vi "Example.vi"() -> ()   [LabVIEW 2019]
uses:
  SubModules/FPGA Addon Speciality IO/Source/Types/PWM.Measure.Digital.Measurement.ctl
  SubModules/FPGA Addon Speciality IO/Source/Types/PWM.Measure.Digital.Result.ctl
  SubModules/FPGA Addon Speciality IO/Source/Types/PWM.Generate.Digital.Convert.Settings.ctl
  SubModules/FPGA Addon Speciality IO/Source/Types/PWM.Generate.Digital.Settings.ctl
  SubModules/FPGA Addon Speciality IO/Source/Types/PWM.Measure.Analog.Measurement.ctl
  SubModules/FPGA Addon Speciality IO/Source/Types/PWM.Measure.Analog.Result.ctl
  SubModules/FPGA Addon Speciality IO/Source/Types/PWM.Measure.Digital.Settings.ctl
  SubModules/FPGA Addon Speciality IO/Source/Types/PWM.Measure.Analog.Settings.ctl
  SubModules/FPGA Addon Speciality IO/Source/Types/Sine.Generate.Settings.ctl
  SubModules/FPGA Addon Speciality IO/Source/Types/Sine.Generate.Convert.Settings.ctl
  <vilib>/Platform/TimedLoop/XDataNode/timing_clust.ctl
  <vilib>/Platform/TimedLoop/XDataNode/nitl_modes.ctl
  <vilib>/Platform/TimedLoop/XDataNode/wakeup.ctl
  <vilib>/Platform/TimedLoop/XDataNode/XDataNode.xnode
  SubModules/FPGA Addon Speciality IO/Source/Speciality FPGA IO.lvlib
  <vilib>/Platform/TimedLoop/XDataNode/XDNodeRunTimeDep.lvlib
panel:
  out "Generation.Sine.Ticks":u32
  in  "Generatie.Sine.Ch1.Settings":T1={"AMP"=10.0, "OFFSET"=0.0, "FREQ"=2000.0}
  in  "Generatie.Sine.Ch0.Settings":T1={"AMP"=1.0, "OFFSET"=0.0, "FREQ"=1000.0}
  out "Generate.Sine.Ch1.Internal.Settings":T2={"AMP"=0.0, "OFFSET"=0.0, "PERIODS/TICKS"=0.0002500000409781933}
  out "Generate.Sine.Chl0.Internal.Settings":T2={"AMP"=0.0, "OFFSET"=0.0, "PERIODS/TICKS"=0.0002500000409781933}
  out "Generate.Sine.Convert.Ticks":u32=84
  in  "Sine":bool=TRUE
  out "PWM1":fxp<+/-,32,8>=11.7987060546875
  out "PWM0":fxp<+/-,32,8>=-12.2012939453125
  out "Generate.Digital.Ticks":u32=114
  out "Measure.Digital.Ticks":u32=84
  out "Measure.Analog.Ticks":u32=84
  in  "Measure.Analog.Ch1.Settings":T3={"ACTIVE EDGE"=FALSE, "TIMEOUT"=40000000, "THRESHOLD"=95.0}
  in  "Measure.Analog.Ch0.Settings":T3={"ACTIVE EDGE"=TRUE, "TIMEOUT"=40000000, "THRESHOLD"=0.0}
  in  "Measure.Digital.Ch1.Settings":T4={"ACTIVE EDGE"=FALSE, "TIMEOUT"=40000000}
  in  "Measure.Digital.Ch0.Settings":T4={"ACTIVE EDGE"=TRUE, "TIMEOUT"=40000000}
  out "Measure.Analog.Analyzed":T5[](array[typedef])=[{"FREQ"=5000.0, "PERIOD"=0.00020000001, "DC"=50.0, "ACTIVE TIME"=0.000100000005, "ACTIVE VOLTAGE"=4.979252, "INACTIVE VOLTAGE"=-4.9794044}, {"FREQ"=999.99994, "PERIOD"=0.001, "DC"=90.0, "ACTIVE TIME"=0.0009, "ACTIVE VOLTAGE"=-6.998723, "INACTIVE VOLTAGE"=6.9985094}]
  out "Measure.Analog.Ch1.Results":T6={"ACTIVE TICKS"=90, "INACTIVE TICKS"=10, "ACQ TICKS"=400, "ACTIVE VOLTAGE"=-6.998723030090332, "INACTIVE VOLTAGE"=6.998509407043457}
  out "Measure.Analog.Ch0.Results":T6={"ACTIVE TICKS"=10, "INACTIVE TICKS"=10, "ACQ TICKS"=400, "ACTIVE VOLTAGE"=4.979251861572266, "INACTIVE VOLTAGE"=-4.979404449462891}
  out "Generate.Digital.Ch1.Internal.Settings":T7={"ACTIVE EDGE"=FALSE, "ACTIVE TICKS"=60000000, "INACTIVE TICKS"=20000000}
  out "Generate.Digital.Ch0.Internal.Settings":T7={"ACTIVE EDGE"=TRUE, "ACTIVE TICKS"=4000, "INACTIVE TICKS"=12000}
  in  "Generate.Digital.Channel0.Settings":T8={"ACTIVE EDGE"=FALSE, "FREQ"=0.5, "DC"=50.0}
  in  "Generate.Digital.Channel0.Settings":T8={"ACTIVE EDGE"=TRUE, "FREQ"=2500.0, "DC"=25.0}
  out "Measure.Digital.Analyzed":T9[](array[typedef])=[{"FREQ"=2500.0, "PERIOD"=0.00040000002, "DC"=25.0, "ACTIVE TIME"=0.000100000005}, {"FREQ"=0.0, "PERIOD"=0.0, "DC"=0.0, "ACTIVE TIME"=0.0}]
  out "Measure.Digital.Ch1.Results":T10
  out "Measure.Digital.Ch0.Results":T10={"ACTIVE TICKS"=4000, "INACTIVE TICKS"=12000, "ACQ TICKS"=1}
  in  "Generation.Sine.Ticks":u32=10 caption="Loop Rate"
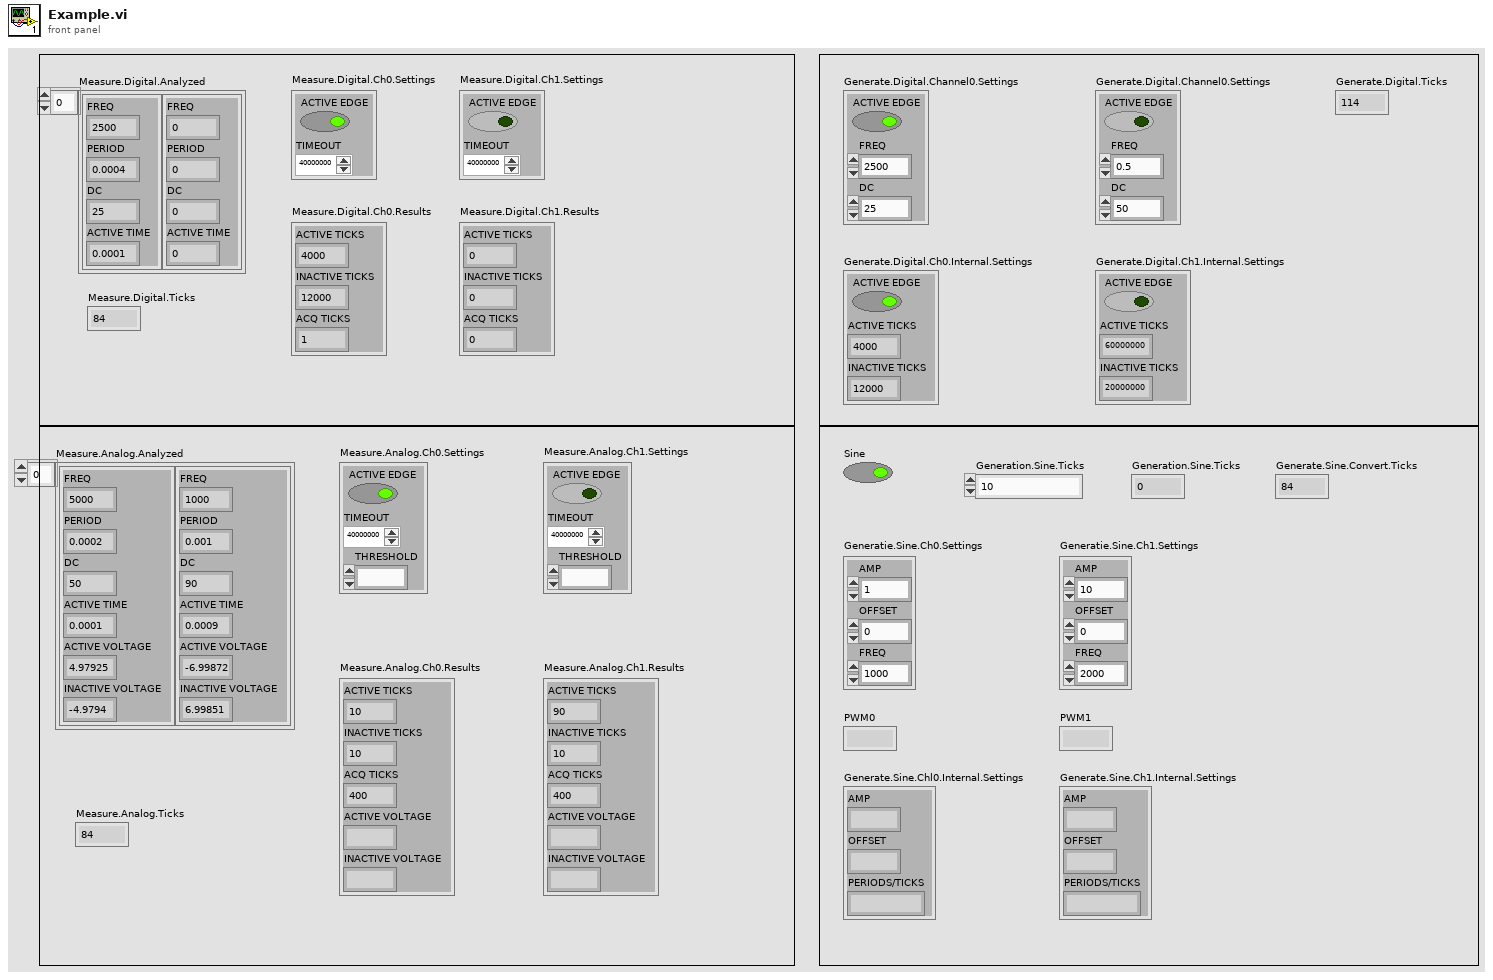
[diagram p1: front panel]
types:
  T1 = typedef "Speciality FPGA IO.lvlib/Sine.Generate.Convert.Settings.ctl" = cluster{"AMP":sgl, "OFFSET":sgl, "FREQ":sgl}
  T2 = typedef "Speciality FPGA IO.lvlib/Sine.Generate.Settings.ctl" = cluster{"AMP":fxp<+/-,32,8>, "OFFSET":fxp<+/-,32,8>, "PERIODS/TICKS":fxp<+,32,0>}
  T3 = typedef "Speciality FPGA IO.lvlib/PWM.Measure.Analog.Settings.ctl" = cluster{"ACTIVE EDGE":bool, "TIMEOUT":u32, "THRESHOLD":fxp<+/-,32,8>}
  T4 = typedef "Speciality FPGA IO.lvlib/PWM.Measure.Digital.Settings.ctl" = cluster{"ACTIVE EDGE":bool, "TIMEOUT":u32}
  T5 = typedef "Speciality FPGA IO.lvlib/PWM.Measure.Analog.Result.ctl" = cluster{"FREQ":sgl, "PERIOD":sgl, "DC":sgl, "ACTIVE TIME":sgl, "ACTIVE VOLTAGE":sgl, "INACTIVE VOLTAGE":sgl}
  T6 = typedef "Speciality FPGA IO.lvlib/PWM.Measure.Analog.Measurement.ctl" = cluster{"ACTIVE TICKS":u32, "INACTIVE TICKS":u32, "ACQ TICKS":u32, "ACTIVE VOLTAGE":fxp<+/-,32,8>, "INACTIVE VOLTAGE":fxp<+/-,32,8>}
  T7 = typedef "Speciality FPGA IO.lvlib/PWM.Generate.Digital.Settings.ctl" = cluster{"ACTIVE EDGE":bool, "ACTIVE TICKS":u32, "INACTIVE TICKS":u32}
  T8 = typedef "Speciality FPGA IO.lvlib/PWM.Generate.Digital.Convert.Settings.ctl" = cluster{"ACTIVE EDGE":bool, "FREQ":sgl, "DC":sgl}
  T9 = typedef "Speciality FPGA IO.lvlib/PWM.Measure.Digital.Result.ctl" = cluster{"FREQ":sgl, "PERIOD":sgl, "DC":sgl, "ACTIVE TIME":sgl}
  T10 = typedef "Speciality FPGA IO.lvlib/PWM.Measure.Digital.Measurement.ctl" = cluster{"ACTIVE TICKS":u32, "INACTIVE TICKS":u32, "ACQ TICKS":u32}
  T11 = typedef "XDNodeRunTimeDep.lvlib/timing_clust.ctl" = cluster{"Expected End [f-1]":u64, "Actual End [f-1]":u64, "Finished Late? [f-1]":bool, "Expected End [i-1]":u64, "Actual End [i-1]":u64, "Finished Late? [i-1]":bool, "Expected Start [i]":u64, "Actual Start [i]":u64, "Expected Start [f]":u64, "Actual Start [f]":u64, "Source Name":string, "Structure Name":string, "Period":i64, "Deadline":i64, "Offset":i64, "Start":i64, "Priority":i32, "Timeout":i32, "Mode":T12, "Wakeup Reason":T13, "Error":errorcluster, "Source Type":string, "Secondary Source Type":string, "Global End Time":u64, "Global Start Time":u64, "Frame Duration":u64, "Iteration Duration":u64, "Assigned CPU":i32, "I/O Scan Engine Mode":u32}
  T12 = typedef "XDNodeRunTimeDep.lvlib/nitl_modes.ctl" = enum32{"No Change", "Process missed periods, maintain original phase", "Discard missed periods, maintain original phase", "Process missed periods, ignore original phase", "Discard missed periods, ignore original phase"}
  T13 = typedef "XDNodeRunTimeDep.lvlib/wakeup.ctl" = enum32{"Normal", "Aborted", "Asynchronous wakeup", "Timing source error", "Timed loop error", "Timeout"}
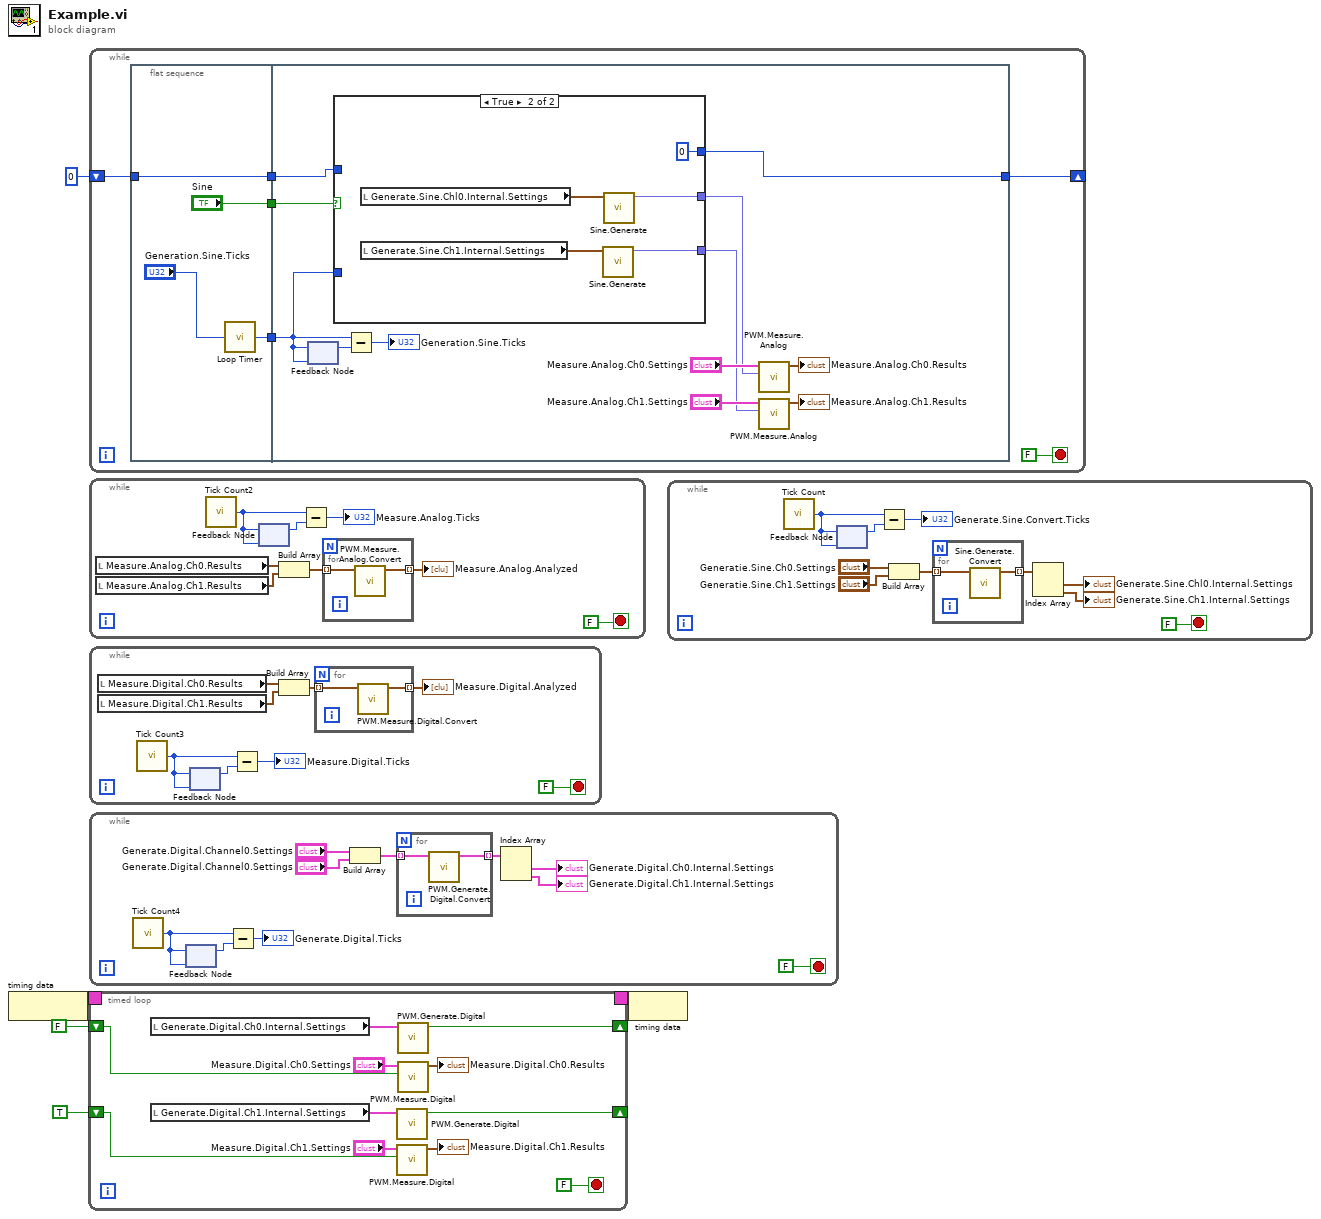
[diagram p0: block diagram]
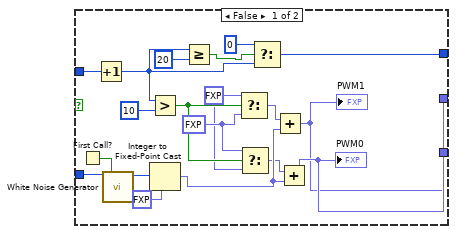
[diagram p2: hidden frame]
diagram:
  n1 = node-c288() -> (w5:T11)
  n2 = timed-loop {
    timing: w5 -> [_]
    timing-out: [_] -> w4
    shift-right: [w15] -> _
    shift-left: TRUE ("Output") -> [w14]
    shift-right: [w13] -> _
    shift-left: FALSE ("Output") -> [w12]
    stop <- FALSE stop-if-true
    n3 = local read "Generate.Digital.Ch0.Internal.Settings"() -> (w9:T7)
    n4 = local read "Generate.Digital.Ch1.Internal.Settings"() -> (w8:T7)
    n5 = call "PWM.Generate.Digital.vi"("Settings"=w8) -> ("Output"=w15:bool)  [unwired: 10 in]
    n6 = call "PWM.Measure.Digital.vi"("State"=w14, "Settings"="Measure.Digital.Ch1.Settings") -> ("Measurement"=→"Measure.Digital.Ch1.Results":T10)  [unwired: 8 in, 1 out]
    n7 = call "PWM.Generate.Digital.vi"("Settings"=w9) -> ("Output"=w13:bool)  [unwired: 10 in]
    n8 = call "PWM.Measure.Digital.vi"("State"=w12, "Settings"="Measure.Digital.Ch0.Settings") -> ("Measurement"=→"Measure.Digital.Ch0.Results":T10)  [unwired: 8 in, 1 out]
  }
  n9 = while {
    shift-right: [w22] -> _
    shift-left: i16 0 -> [w23]
    stop <- FALSE stop-if-true
    n10 = flat-sequence {
      tunnel: [w27] -> w24
      tunnel: w23 -> [w27]
      tunnel: [w26] -> w21
      tunnel: ["Sine"] -> w19
      tunnel: w24 -> [w33]
      tunnel: [w34] -> w22
      tunnel: w21 -> [w31]
      tunnel: w19 -> [w32]
      frame #0 {
        n11 = call "Loop Timer"("Count(uSec)"="Generation.Sine.Ticks") -> ("Tick Count(uSec)"=w26:u32)
      }
      frame #1 {
        n12 = feedback-in #1(w31) -> ()
        n13 = feedback #1(w31) -> (w30:u32)
        n14 = case shown="True" w32 {
          tunnel: [w41 w63] -> w36
          tunnel: [w42 w62] -> w35
          tunnel: w33 -> [w45 _]
          tunnel: w31 -> [w44 _]
          tunnel: [w43 i16 0 ("t")] -> w34
          frame False {
            w53 = fxp<+/-,32,8> 12.0 ("t")
            w54 = fxp<+/-,32,8> -12.0 ("PWM")
            n15 = First Call?() -> (First Call?: T/F=w52:bool)
            n16 = Increment(x=w45) -> (x+1=w56:i16)
            n17 = call "White Noise Generator"("seed"=w44, "reset"=w52) -> ("white noise out"=w51:i16)  [unwired: 13 in]
            n18 = Greater?(x=w56, y=i16 10) -> (0:w55:bool)
            n19 = Integer to Fixed-Point Cast(fixed-point type=fxp<+/-,16,1> 0.0, integer=w51) -> (fixed-point=w49:fxp<+/-,16,1>)
            n20 = Greater Or Equal?(x=w56, y=i16 20) -> (x >= y?=w46:bool)
            n21 = Select(t=w53, s=w55, f=w54) -> (s? t:f=w47:fxp<+/-,32,8>)
            n22 = Select(t=w54, s=w55, f=w53) -> (s? t:f=w48:fxp<+/-,32,8>)
            n23 = Select(t=i16 0, s=w46, f=w56) -> (s? t:f=w43:i16)
            n24 = Add(x=w47, y=w49) -> (x+y=w41:fxp<+/-,33,9>)
            "PWM1" <- w41
            n25 = Add(x=w48, y=w49) -> (x+y=w42:fxp<+/-,33,9>)
            "PWM0" <- w42
          }
          frame True {
            n26 = local read "Generate.Sine.Chl0.Internal.Settings"() -> (w61:T2)
            n27 = local read "Generate.Sine.Ch1.Internal.Settings"() -> (w60:T2)
            n28 = call "Sine.Generate.vi"("Settings"=w60) -> ("Output"=w63:fxp<+/-,32,8>)  [unwired: 10 in]
            n29 = call "Sine.Generate.vi"("Settings"=w61) -> ("Output"=w62:fxp<+/-,32,8>)  [unwired: 10 in]
          }
        }
        n30 = Subtract(x=w31, y=w30) -> (x-y=→"Generation.Sine.Ticks":u32)
        n31 = call "PWM.Measure.Analog.vi"("PWM"=w35, "Settings"="Measure.Analog.Ch0.Settings") -> ("Measurement"=→"Measure.Analog.Ch0.Results":T6)  [unwired: 8 in, 1 out]
        n32 = call "PWM.Measure.Analog.vi"("PWM"=w36, "Settings"="Measure.Analog.Ch1.Settings") -> ("Measurement"=→"Measure.Analog.Ch1.Results":T6)  [unwired: 8 in, 1 out]
      }
    }
  }
  n33 = while {
    stop <- FALSE stop-if-true
    n34 = local read "Measure.Analog.Ch0.Results"() -> (w71:T6)
    n35 = local read "Measure.Analog.Ch1.Results"() -> (w70:T6)
    n36 = call "Tick Count2"() -> ("Tick Count(Ticks)"=w65:u32)
    n37 = feedback #2(w65) -> (w67:u32)
    n38 = feedback-in #2(w65) -> ()
    n39 = Build Array(w71, w70) -> (w69:T6[])
    n40 = Subtract(x=w65, y=w67) -> (x-y=→"Measure.Analog.Ticks":u32)
    n41 = for {
      tunnel: [w74] -> w68 mode=indexing
      tunnel: w69 -> [w73] mode=indexing
      n42 = call "PWM.Measure.Analog.Convert.vi"("Measurement"=w73) -> ("Result"=w74:T5)  [unwired: 10 in]
    }
    "Measure.Analog.Analyzed" <- w68
  }
  n43 = while {
    stop <- FALSE stop-if-true
    n44 = local read "Measure.Digital.Ch0.Results"() -> (w80:T10)
    n45 = local read "Measure.Digital.Ch1.Results"() -> (w81:T10)
    n46 = call "Tick Count3"() -> ("Tick Count(Ticks)"=w77:u32)
    n47 = feedback #3(w77) -> (w75:u32)
    n48 = feedback-in #3(w77) -> ()
    n49 = Subtract(x=w77, y=w75) -> (x-y=→"Measure.Digital.Ticks":u32)
    n50 = Build Array(w80, w81) -> (w79:T10[])
    n51 = for {
      tunnel: w79 -> [w84] mode=indexing
      tunnel: [w83] -> w78 mode=indexing
      n52 = call "PWM.Measure.Digital.Convert.vi"("Measurement"=w84) -> ("Result"=w83:T9)  [unwired: 10 in]
    }
    "Measure.Digital.Analyzed" <- w78
  }
  n53 = while {
    stop <- FALSE stop-if-true
    n54 = call "Tick Count4"() -> ("Tick Count(Ticks)"=w85:u32)
    n55 = feedback #4(w85) -> (w87:u32)
    n56 = feedback-in #4(w85) -> ()
    n57 = Subtract(x=w85, y=w87) -> (x-y=→"Generate.Digital.Ticks":u32)
    n58 = Build Array("Generate.Digital.Channel0.Settings", "Generate.Digital.Channel0.Settings") -> (w91:T8[])
    n59 = for {
      tunnel: [w96] -> w90 mode=indexing
      tunnel: w91 -> [w95] mode=indexing
      n60 = call "PWM.Generate.Digital.Convert.vi"("Settings"=w95) -> ("Settings"=w96:T7)  [unwired: 10 in]
    }
    n61 = Index Array(array=w90) -> (element #1=→"Generate.Digital.Ch0.Internal.Settings":T7, element #2=→"Generate.Digital.Ch1.Internal.Settings":T7)  [unwired: 2 in]
  }
  n62 = node-c288(w4) -> ()
  n63 = while {
    stop <- FALSE stop-if-true
    n64 = call "Tick Count"() -> ("Tick Count(Ticks)"=w102:u32)
    n65 = feedback #5(w102) -> (w104:u32)
    n66 = feedback-in #5(w102) -> ()
    n67 = Subtract(x=w102, y=w104) -> (x-y=→"Generate.Sine.Convert.Ticks":u32)
    n68 = Build Array("Generatie.Sine.Ch0.Settings", "Generatie.Sine.Ch1.Settings") -> (w105:T1[])
    n69 = for {
      tunnel: [w108] -> w101 mode=indexing
      tunnel: w105 -> [w107] mode=indexing
      n70 = call "Sine.Generate.Convert.vi"("Settings"=w107) -> ("Settings"=w108:T2)  [unwired: 10 in]
    }
    n71 = Index Array(array=w101) -> (element #1=→"Generate.Sine.Chl0.Internal.Settings":T2, element #2=→"Generate.Sine.Ch1.Internal.Settings":T2)  [unwired: 2 in]
  }
